vi "电流加载及换向回读-PLC（S200Smart）.vi"(0 "6510 in":refnum<visa-resource-name>, 1 "TDK in":refnum<visa-resource-name>, 2 "输入电流":dbl, 3 "Delay Time (s)":dbl=1.0 caption="延迟时间(s)", 4 "电源台数":u8=1, 5 "error in":errorcluster, 6 "引用输出":refnum<k24>, 7 "y":dbl=5000.0 format="%#_13g") -> (14 "2700 out":refnum<visa-resource-name>, 15 "TDK out":refnum<visa-resource-name>, 16 "实际电流":dbl, 19 "error out":errorcluster)   [LabVIEW 2021]
uses:
  <instrlib>/Keithley 27XX/Public/Data/Read Single Point.vi
  <instrlib>/TDK-Lambda G Series/TDK-Lambda G Series.lvlib
  <instrlib>/Keithley 27XX/Keithley 27XX.lvlib
panel:
  out "x*y":dbl
  # "TDK 电流加载及换向"
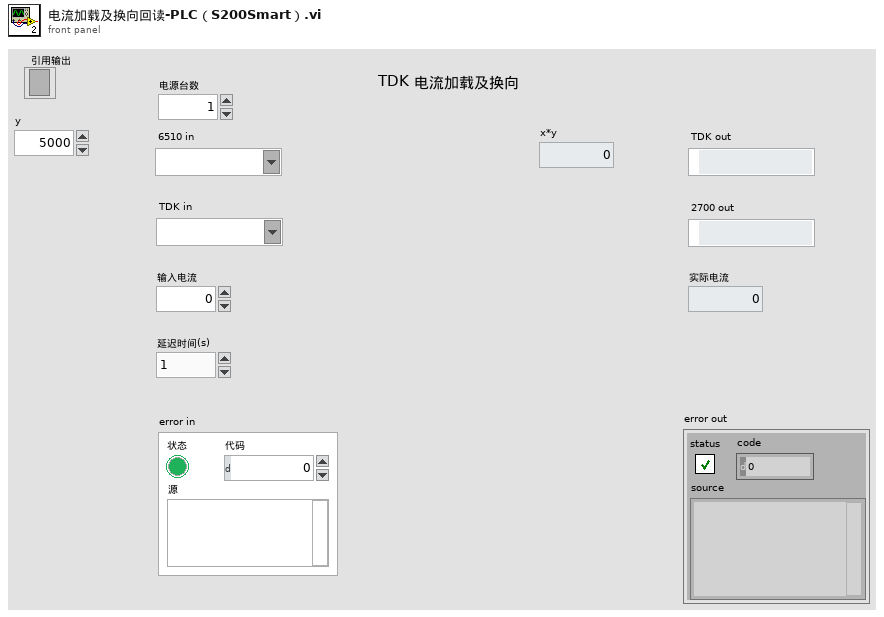
[diagram p1: front panel]
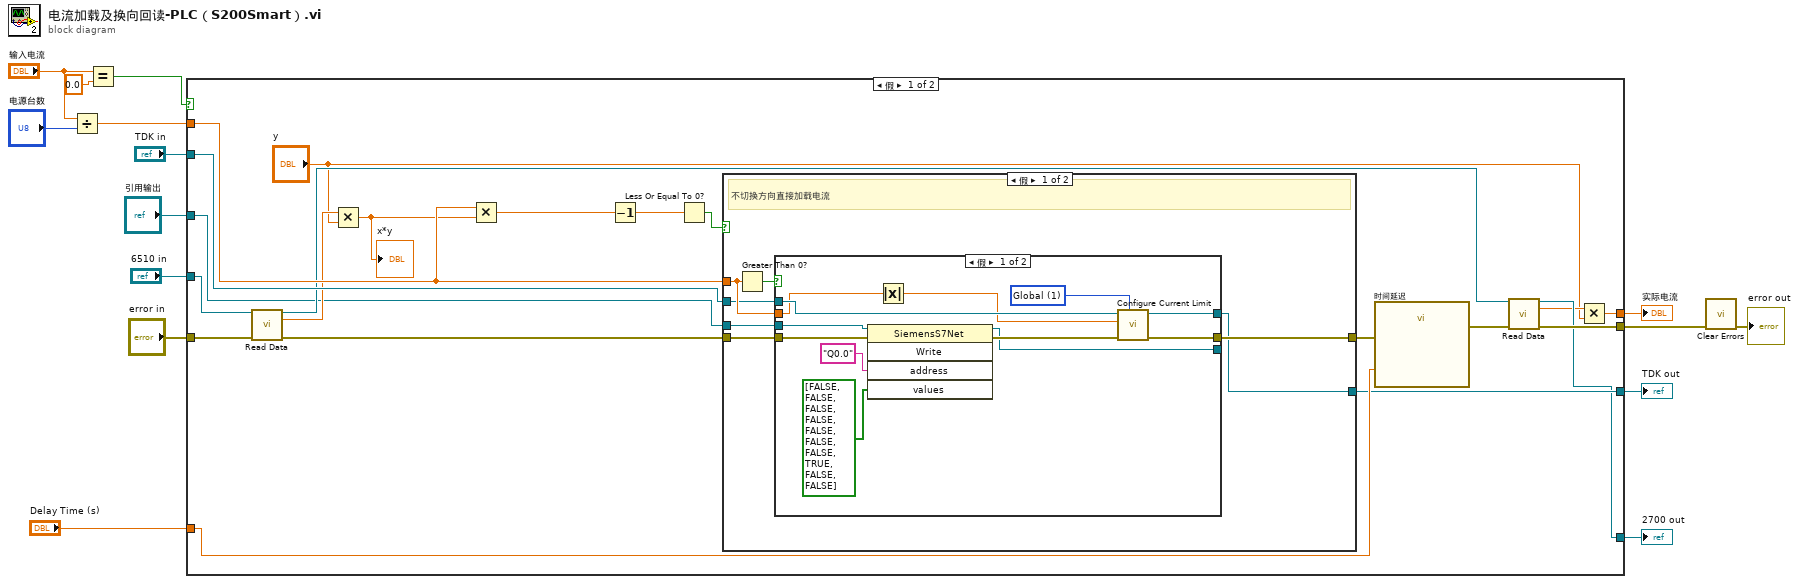
[diagram p0: block diagram]
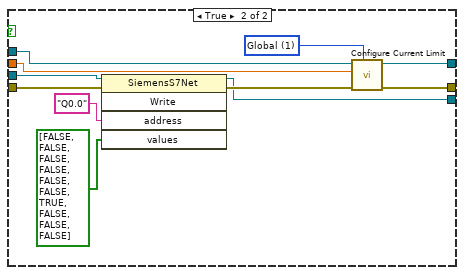
[diagram p2: hidden frame]
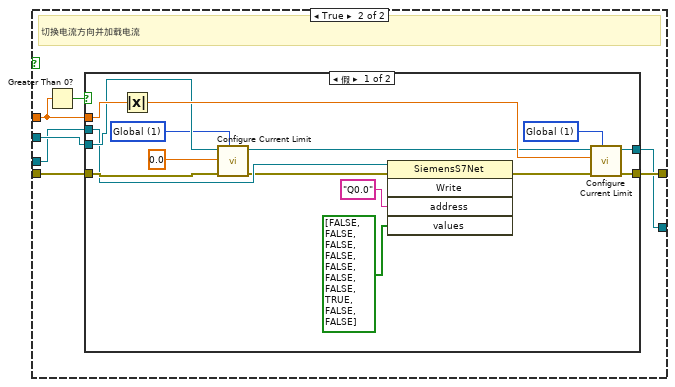
[diagram p3: hidden frame]
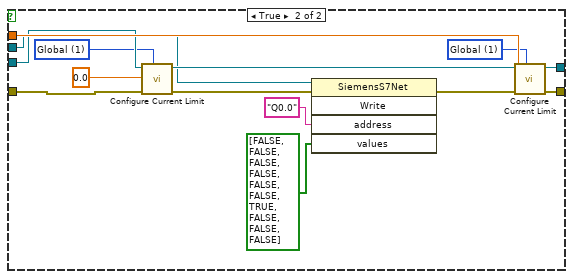
[diagram p4: hidden frame]
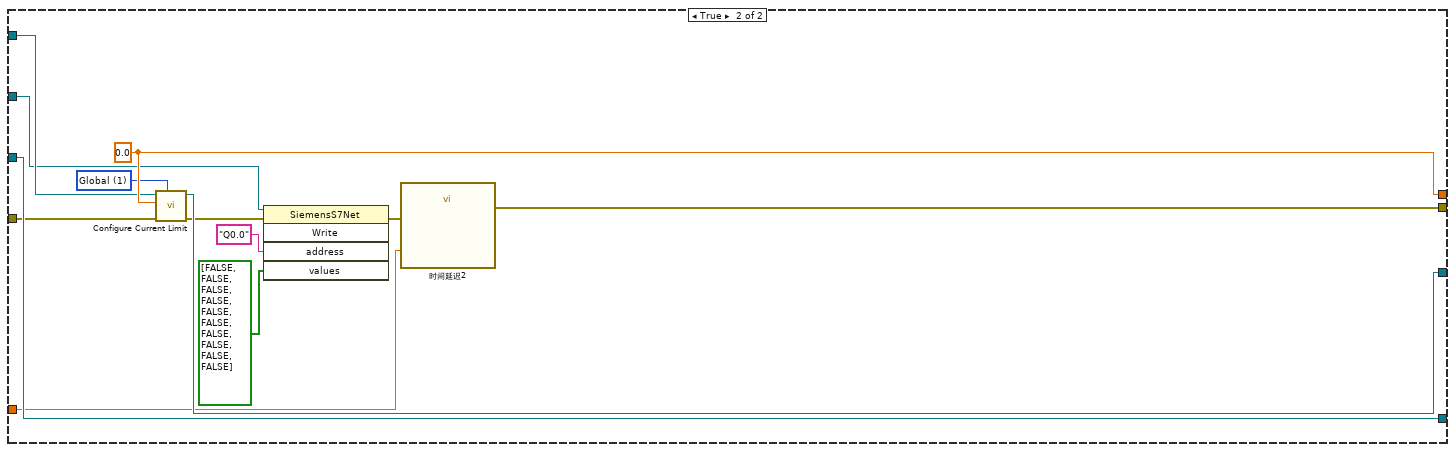
[diagram p5: hidden frame]
diagram:
  n1 = Divide(x="输入电流", y="电源台数") -> (x/y=w5:dbl)
  n2 = Equal?(x="输入电流", y=0.0) -> (x = y?=w11:bool)
  n3 = case shown="假" w11 {
    tunnel: "TDK in" -> [w33 w111]
    tunnel: [w20 w109] -> w1
    tunnel: "Delay Time (s)" -> [w31 w108]
    tunnel: "error in" -> [w24 w113]
    tunnel: [w30 w114] -> w13
    tunnel: "6510 in" -> [w25 w115]
    tunnel: [w19 w115] -> w9
    tunnel: w5 -> [w29 _]
    tunnel: [w27 w112] -> w10
    tunnel: "引用输出" -> [w16 w105]
    frame False {
      n4 = call-poly <instrlib>:"Read Data.vi"("VISA resource name"=w25, "error in (no error)"=w24) -> ("VISA resource name out"=w22:refnum<visa-resource-name>, "Measurement Data"=w26:dbl, "error out"=w23:errorcluster)  [unwired: 11 in]
      n5 = Multiply(x=w26, y="y") -> (x*y=w28:dbl)
      "x*y" <- w28
      n6 = Multiply(x=w29, y=w28) -> (x*y=w35:dbl)
      n7 = Decrement(x=w35) -> (x-1=w34:dbl)
      n8 = Less Or Equal To 0?(x=w34) -> (x <= 0?=w36:bool)
      n9 = case shown="假" w36 {
        tunnel: w29 -> [w42 w73]
        tunnel: w23 -> [w39 w69]
        tunnel: w33 -> [w41 w71]
        tunnel: [w40 w70] -> w32
        tunnel: [w38 w68] -> w30
        tunnel: w16 -> [w37 w67]
        frame False {
          # "不切换方向直接加载电流"
          n10 = Greater Than 0?(x=w42) -> (x > 0?=w43:bool)
          n11 = case shown="假" w43 {
            tunnel: w42 -> [w45 w64]
            tunnel: w41 -> [w47 w65]
            tunnel: [w54 w63] -> w40
            tunnel: w39 -> [w46 w61]
            tunnel: [w55 w66] -> w38
            tunnel: [w51 w59] -> _
            tunnel: w37 -> [w48 w56]
            frame False {
              w53 = u16 1 items=["Single", "Global"] ("Globalize (0: Single)")
              n12 = invoke class="SiemensS7Net" method="Write"(reference=w48, error in=w46, "address"="Q0.0", "values"=bool[] [FALSE, FALSE, FALSE, FALSE, FALSE, FALSE, FALSE, TRUE, FALSE, FALSE]) -> (reference out=w51:refnum<k24>, error out=w52:errorcluster)  [unwired: 1 in, 3 out]
              n13 = Absolute Value(x=w45) -> (abs(x)=w44:dbl)
              n14 = call <instrlib>:"Configure Current Limit.vi"("Globalize (0: Single)"=w53, "error in (no error)"=w52, "Current Limit (0A)"=w44, "VISA resource name"=w47) -> ("error out"=w54:errorcluster, "VISA resource name out"=w55:refnum<visa-resource-name>)  [unwired: 6 in]
            }
            frame True {
              w62 = u16 1 items=["Single", "Global"] ("Globalize (0: Single)")
              n15 = invoke class="SiemensS7Net" method="Write"(reference=w56, error in=w61, "address"="Q0.0", "values"=bool[] [FALSE, FALSE, FALSE, FALSE, FALSE, FALSE, TRUE, FALSE, FALSE, FALSE]) -> (reference out=w59:refnum<k24>, error out=w60:errorcluster)  [unwired: 1 in, 3 out]
              n16 = call <instrlib>:"Configure Current Limit.vi"("Globalize (0: Single)"=w62, "error in (no error)"=w60, "Current Limit (0A)"=w64, "VISA resource name"=w65) -> ("error out"=w63:errorcluster, "VISA resource name out"=w66:refnum<visa-resource-name>)  [unwired: 6 in]
            }
          }
        }
        frame True {
          # "切换电流方向并加载电流"
          n17 = Greater Than 0?(x=w73) -> (x > 0?=w72:bool)
          n18 = case shown="假" w72 {
            tunnel: w73 -> [w88 w100]
            tunnel: w71 -> [w84 w99]
            tunnel: [w87 w102] -> w70
            tunnel: w69 -> [w82 w97]
            tunnel: [w86 w101] -> w68
            tunnel: w67 -> [w79 w89]
            frame False {
              w80 = u16 1 items=["Single", "Global"] ("Globalize (0: Single)")
              w81 = u16 1 items=["Single", "Global"] ("Globalize (0: Single)")
              n19 = Absolute Value(x=w88) -> (abs(x)=w85:dbl)
              n20 = call <instrlib>:"Configure Current Limit.vi"("Globalize (0: Single)"=w80, "error in (no error)"=w82, "Current Limit (0A)"=0.0 ("Curr(0)"), "VISA resource name"=w84) -> ("error out"=w78:errorcluster, "VISA resource name out"=w74:refnum<visa-resource-name>)  [unwired: 6 in]
              n21 = invoke class="SiemensS7Net" method="Write"(reference=w79, error in=w78, "address"="Q0.0", "values"=bool[] [FALSE, FALSE, FALSE, FALSE, FALSE, FALSE, FALSE, TRUE, FALSE, FALSE]) -> (error out=w77:errorcluster)  [unwired: 1 in, 4 out]
              n22 = call <instrlib>:"Configure Current Limit.vi"("Globalize (0: Single)"=w81, "error in (no error)"=w77, "Current Limit (0A)"=w85, "VISA resource name"=w74) -> ("error out"=w87:errorcluster, "VISA resource name out"=w86:refnum<visa-resource-name>)  [unwired: 6 in]
            }
            frame True {
              w94 = u16 1 items=["Single", "Global"] ("Globalize (0: Single)")
              w95 = u16 1 items=["Single", "Global"] ("Globalize (0: Single)")
              n23 = call <instrlib>:"Configure Current Limit.vi"("Globalize (0: Single)"=w94, "error in (no error)"=w97, "Current Limit (0A)"=0.0 ("Curr(0)"), "VISA resource name"=w99) -> ("error out"=w93:errorcluster, "VISA resource name out"=w96:refnum<visa-resource-name>)  [unwired: 6 in]
              n24 = invoke class="SiemensS7Net" method="Write"(reference=w89, error in=w93, "address"="Q0.0", "values"=bool[] [FALSE, FALSE, FALSE, FALSE, FALSE, FALSE, TRUE, FALSE, FALSE, FALSE]) -> (error out=w92:errorcluster)  [unwired: 1 in, 4 out]
              n25 = call <instrlib>:"Configure Current Limit.vi"("Globalize (0: Single)"=w95, "error in (no error)"=w92, "Current Limit (0A)"=w100, "VISA resource name"=w96) -> ("error out"=w102:errorcluster, "VISA resource name out"=w101:refnum<visa-resource-name>)  [unwired: 6 in]
            }
          }
        }
      }
      n26 = call "时间延迟"("error in (no error)"=w32, "Delay Time (s)"=w31) -> ("error out"=w21:errorcluster)  [unwired: 9 in]
      n27 = call-poly <instrlib>:"Read Data.vi"("VISA resource name"=w22, "error in (no error)"=w21) -> ("VISA resource name out"=w19:refnum<visa-resource-name>, "Measurement Data"=w18:dbl, "error out"=w20:errorcluster)  [unwired: 11 in]
      n28 = Multiply(x=w18, y="y") -> (x*y=w27:dbl)
    }
    frame True {
      w110 = u16 1 items=["Single", "Global"] ("Globalize (0: Single)")
      w112 = 0.0 ("Curr(0)")
      n29 = call <instrlib>:"Configure Current Limit.vi"("Globalize (0: Single)"=w110, "error in (no error)"=w113, "Current Limit (0A)"=w112, "VISA resource name"=w111) -> ("error out"=w106:errorcluster, "VISA resource name out"=w114:refnum<visa-resource-name>)  [unwired: 6 in]
      n30 = invoke class="SiemensS7Net" method="Write"(reference=w105, error in=w106, "address"="Q0.0", "values"=bool[] [FALSE, FALSE, FALSE, FALSE, FALSE, FALSE, FALSE, FALSE, FALSE, FALSE]) -> (error out=w107:errorcluster)  [unwired: 1 in, 4 out]
      n31 = call "时间延迟2"("error in (no error)"=w107, "Delay Time (s)"=w108) -> ("error out"=w109:errorcluster)  [unwired: 9 in]
    }
  }
  "实际电流" <- w10
  "TDK out" <- w13
  "2700 out" <- w9
  n32 = call <vilib>:"Clear Errors.vi"("error in (no error)"=w1) -> ("error out"=→"error out":errorcluster)  [unwired: 5 in, 1 out]
